vi "rinse-2_FMI.vi"(7 "RequestedValve#":i32, 8 "Last?":bool, 10 "Strokes":i32=5) -> ()   [LabVIEW 2019]
panel:
  out "xxx":bool[](array[boolean])
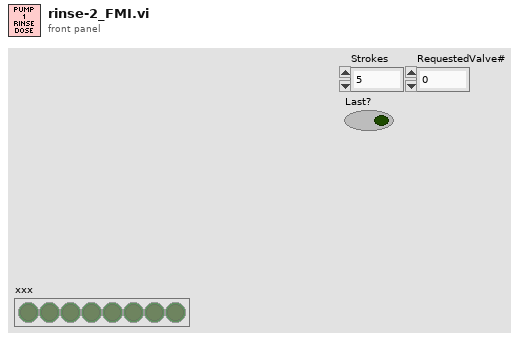
[diagram p1: front panel]
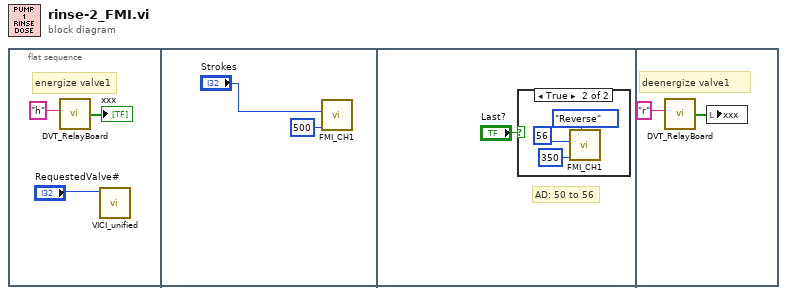
[diagram p0: block diagram]
diagram:
  n1 = flat-sequence {
    frame #0 {
      # "energize valve1"
      n2 = call "DVT_RelayBoard.vi"("write buffer"="h") -> ("Boolean array"=→"xxx":bool[])  [unwired: 3 in, 2 out]
      n3 = call "VICI_unified.vi"("RequestedValve#"="RequestedValve#") -> ()  [unwired: 11 in]
    }
    frame #1 {
      n4 = call "FMI_CH1.vi"("RPM"=500, "Strokes"="Strokes") -> ()  [unwired: 6 in]
    }
    frame #2 {
      # "AD: 50 to 56"
      n5 = case shown="True" "Last?" {
        frame False {
        }
        frame True {
          n6 = call "FMI_CH1.vi"("Direction"=enum16{"Forward", "Reverse"}."Reverse", "RPM"=350, "Strokes"=56 ("Strokes 2")) -> ()  [unwired: 5 in]
        }
      }
    }
    frame #3 {
      # "deenergize valve1"
      n7 = call "DVT_RelayBoard.vi"("write buffer"="r") -> ("Boolean array"=w11:bool[])  [unwired: 3 in, 2 out]
      n8 = local write "xxx"(w11) -> ()
    }
  }
